vi "DSF.Engine.Transceiver Thread.Get Debug Flags.vi"(11 "Transceiver Thread in":refnum<class "DSF.Engine.Transceiver Thread.lvclass">) -> (2 "Debug Flags":refnum<class "DSF.Engine.Debug Flags.lvclass">, 3 "Transceiver Thread out":refnum<class "DSF.Engine.Transceiver Thread.lvclass">)   [LabVIEW 2017, in "DSF.Engine.lvlib" / "DSF.Engine.Transceiver Thread.lvclass"]
uses:
  DSF.Engine.Transceiver Thread.lvclass
  Debug/DSF.Engine.Debug Flags.lvclass
  DSF.Engine.Transceiver Thread.lvclass/DSF.Engine.Transceiver Thread.ctl
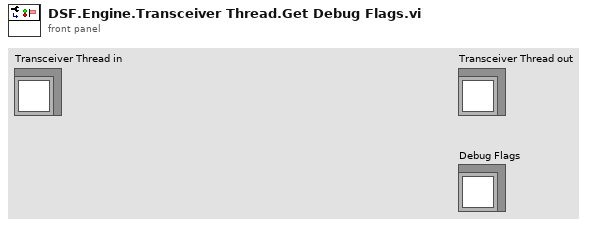
[diagram p1: front panel]
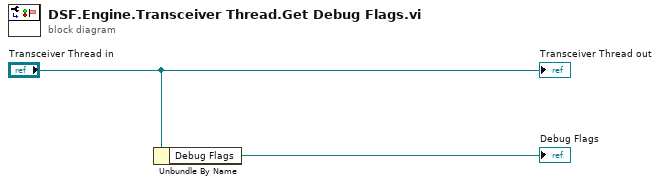
[diagram p0: block diagram]
diagram:
  n1 = Unbundle By Name("Transceiver Thread in") -> ("Debug Flags"=→"Debug Flags":refnum<class "DSF.Engine.Debug Flags.lvclass">)
  "Transceiver Thread out" <- "Transceiver Thread in"
